vi "RPM_Math.vi"(11 "Velocity in":dbl) -> (3 "RPM":dbl)   [LabVIEW 2019]
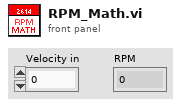
[diagram p1: front panel]
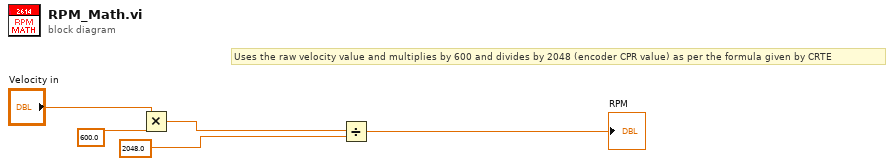
[diagram p0: block diagram]
diagram:
  # "Uses the raw velocity value and multiplies by 600 and divides by 2048 (encoder CPR value) as per the formula given by CRTE"
  n1 = Multiply(x="Velocity in", y=600.0) -> (x*y=w3:dbl)
  n2 = Divide(x=w3, y=2048.0) -> (x/y=→"RPM":dbl)
